vi "Simple SeqProcessor.vi"() -> ()   [LabVIEW 2016, in "SeqProcessor.lvlib"]
uses:
  SeqProcessor.lvlib
  controls/StepScript.ctl
  controls/StepType.ctl
  controls/StepResult.ctl
  controls/StepStatus.ctl
  <vilib>/addons/Qbus/Qbus.lvclass
panel:
  out "error out (no error)":errorcluster
  in  "error in (no error)":errorcluster
  in  "Seq":T1[](array[typedef])=[{"Type"=enum."Normal", "Step"=[{"Action"="StepA", "Process"="ProcessB", "Jump"=0, "Data"="", "Condition"=FALSE}]}, {"Type"=enum."Normal", "Step"=[{"Action"="StepB", "Process"="ProcessB", "Jump"=0, "Data"="", "Condition"=FALSE}]}, {"Type"=enum."Normal", "Step"=[{"Action"="StepC", "Process"="ProcessA", "Jump"=0, "Data"="", "Condition"=FALSE}]}]
  in  "Run":bool
  in  "Stop":bool
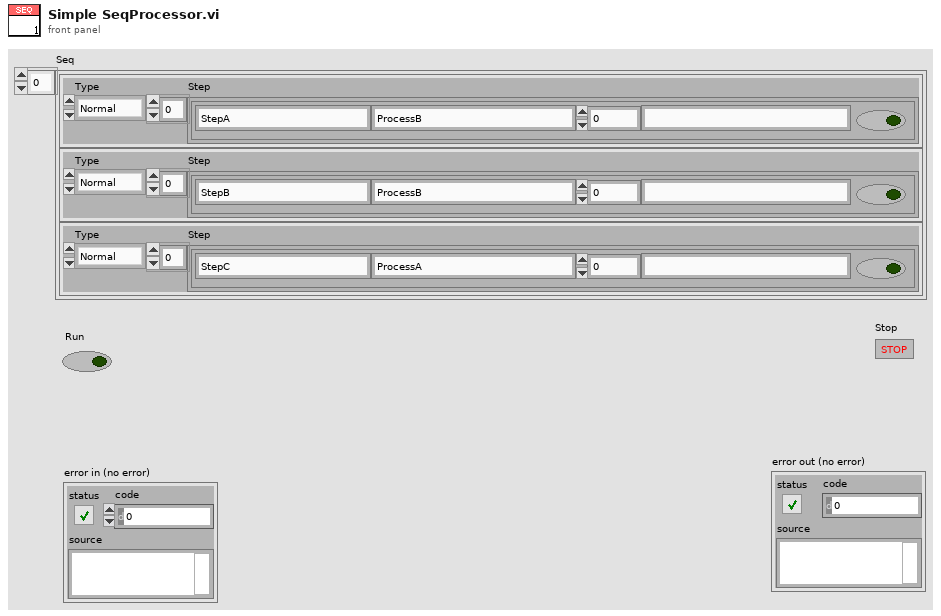
[diagram p1: front panel]
types:
  T1 = typedef "SeqProcessor.lvlib/StepScript.ctl" = cluster{"Type":T2, "Step":cluster{"Action":string, "Process":string, "Jump":i32, "Data":string, "Condition":bool}[]}
  T2 = typedef "SeqProcessor.lvlib/StepType.ctl" = enum16{"Normal", "Parallel", "Conditional", "Jump"}
  T3 = typedef "SeqProcessor.lvlib/StepResult.ctl" = cluster{"Status":T4, "Message":string, "Data":variant}
  T4 = typedef "SeqProcessor.lvlib/StepStatus.ctl" = enum16{"Undone", "Finish", "Error"}
  T5 = typedef "SeqProcessor.lvlib/StepIndex.ctl" = cluster{"Index1":u32, "Index2":u32}
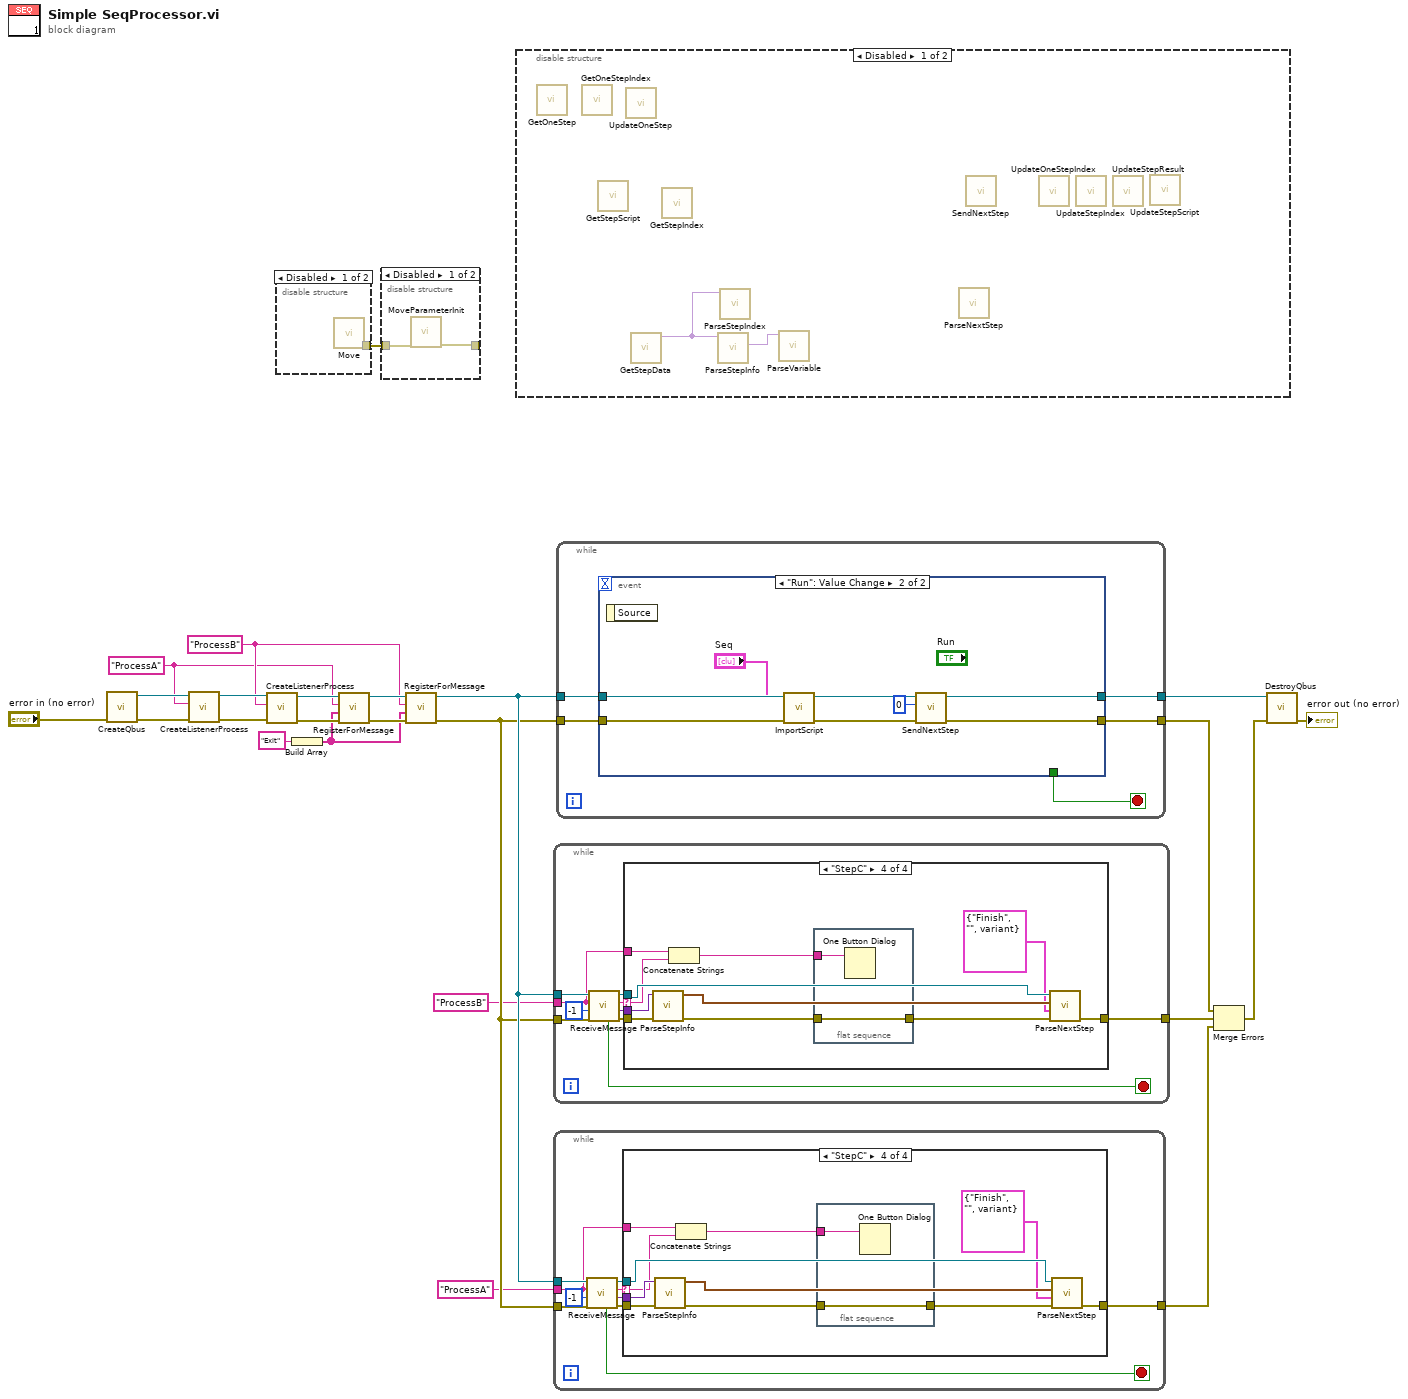
[diagram p0: block diagram]
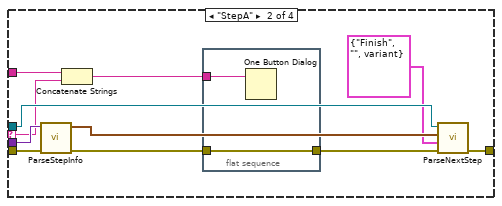
[diagram p3: hidden frame]
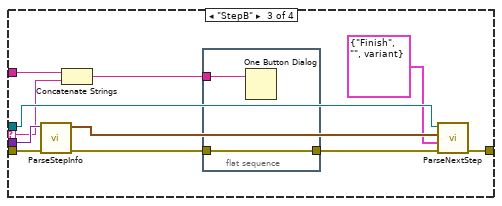
[diagram p4: hidden frame]
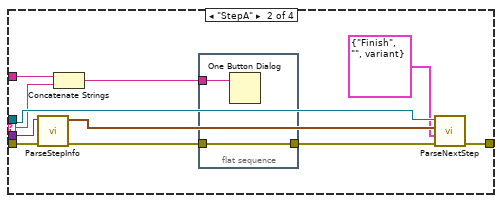
[diagram p6: hidden frame]
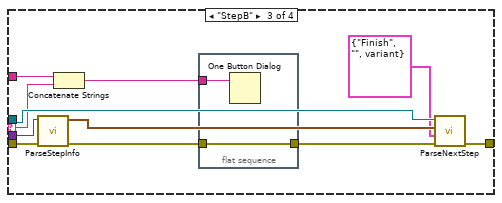
[diagram p7: hidden frame]
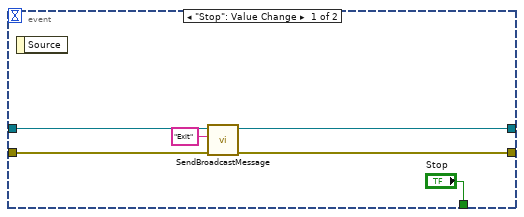
[diagram p8: hidden frame]
diagram:
  w8 = "ProcessB" ("process name")
  w6 = "ProcessA" ("process name")
  n1 = call <vilib>:"CreateQbus.vi"("error in (no error)"="error in (no error)") -> ("error out"=w22:errorcluster, "Qbus"=w23:refnum<class "Qbus.lvclass">)  [unwired: 9 in]
  n2 = call <vilib>:"CreateListenerProcess.vi"("error in (no error)"=w22, "process name"=w6, "Qbus in"=w23) -> ("error in (no error)"=w21:errorcluster, "Qbus out"=w20:refnum<class "Qbus.lvclass">)  [unwired: 7 in]
  n3 = call <vilib>:"CreateListenerProcess.vi"("error in (no error)"=w21, "process name"=w8, "Qbus in"=w20) -> ("error in (no error)"=w15:errorcluster, "Qbus out"=w16:refnum<class "Qbus.lvclass">)  [unwired: 7 in]
  n4 = disable-structure shown="Disabled" {
    disable-tunnel: [w25 _] -> w24
    frame Disabled {
      n5 = call "Move.vi"() -> ("error out"=w25:errorcluster)  [unwired: 11 in]
    }
    frame Enabled {
    }
  }
  n6 = Build Array("Exit" ("message name")) -> (w9:string[])
  n7 = call <vilib>:"RegisterForMessage.vi"("error in (no error)"=w15, "message names"=w9, "process name"=w6, "Qbus in"=w16) -> ("error in (no error)"=w13:errorcluster, "Qbus out"=w14:refnum<class "Qbus.lvclass">)  [unwired: 6 in]
  n8 = disable-structure shown="Disabled" {
    disable-tunnel: w24 -> [w27 w28]
    disable-tunnel: [w26 w28] -> _
    frame Disabled {
      n9 = call "MoveParameterInit.vi"("error in (no error)"=w27) -> ("Error Out"=w26:errorcluster)  [unwired: 10 in]
    }
    frame Enabled {
    }
  }
  n10 = call <vilib>:"RegisterForMessage.vi"("error in (no error)"=w13, "message names"=w9, "process name"=w8, "Qbus in"=w14) -> ("error in (no error)"=w11:errorcluster, "Qbus out"=w12:refnum<class "Qbus.lvclass">)  [unwired: 6 in]
  n11 = disable-structure shown="Disabled" {
    frame Disabled {
      n12 = call "GetOneStep.vi"() -> ()  [unwired: 9 in, 3 out]
      n13 = call "GetOneStepIndex.vi"() -> ()  [unwired: 9 in, 3 out]
      n14 = call "GetStepScript.vi"() -> ()  [unwired: 9 in, 3 out]
      n15 = call "UpdateOneStep.vi"() -> ()  [unwired: 11 in, 1 out]
      n16 = call "GetStepData.vi"() -> ("Data"=w29:variant)  [unwired: 9 in, 2 out]
      n17 = call "GetStepIndex.vi"() -> ()  [unwired: 9 in, 3 out]
      n18 = call "ParseStepInfo.vi"("Data"=w29) -> ("StepData"=w30:variant)  [unwired: 7 in, 3 out]
      n19 = call "ParseStepIndex.vi"("Data"=w29) -> ()  [unwired: 9 in, 2 out]
      n20 = call "ParseVariable.vi"("Variant"=w30) -> ()  [unwired: 8 in, 3 out]
      n21 = call "ParseNextStep.vi"() -> ()  [unwired: 11 in, 1 out]
      n22 = call "SendNextStep.vi"() -> ()  [unwired: 11 in, 1 out]
      n23 = call "UpdateOneStepIndex.vi"() -> ()  [unwired: 9 in, 3 out]
      n24 = call "UpdateStepIndex.vi"() -> ()  [unwired: 11 in, 1 out]
      n25 = call "UpdateStepResult.vi"() -> ()  [unwired: 10 in, 2 out]
      n26 = call "UpdateStepScript.vi"() -> ()  [unwired: 11 in, 1 out]
    }
    frame Enabled {
    }
  }
  n27 = while {
    tunnel: w12 -> [w39]
    tunnel: w11 -> [w40]
    tunnel: "ProcessB" ("process name") -> [w31]
    tunnel: [w32] -> w18
    stop <- w34 stop-if-true
    n28 = call <vilib>:"ReceiveMessage.vi"("error in (no error)"=w40, "timeout (0)"=-1, "process name"=w31, "Qbus in"=w39) -> ("error in (no error)"=w35:errorcluster, "message value"=w36:variant, "message name"=w37:string, "Qbus out"=w38:refnum<class "Qbus.lvclass">, "exit"=w34:bool)  [unwired: 2 in, 1 out]
    n29 = case shown="\"StepC\"" w37 {
      selector: w37 -> [_ w45 w58 w71]
      tunnel: w38 -> [_ w49 w62 w75]
      tunnel: w36 -> [_ w51 w64 w77]
      tunnel: w35 -> [w41 w52 w65 w78]
      tunnel: [w41 w48 w61 w74] -> w32
      tunnel: w31 -> [_ w46 w59 w72]
      frame "", Default {
      }
      frame "StepA" {
        n30 = call "ParseStepInfo.vi"("error in (no error)"=w52, "Data"=w51) -> ("error out"=w43:errorcluster, "StepIndex"=w50:T5)  [unwired: 6 in, 2 out]
        n31 = Concatenate Strings(w46, w45) -> (w44:string)
        n32 = flat-sequence {
          tunnel: w44 -> [w54]
          tunnel: w43 -> [w53]
          tunnel: [w53] -> w42
          frame #0 {
            n33 = One Button Dialog(message=w54) -> ()  [unwired: 1 in, 1 out]
          }
        }
        n34 = call "ParseNextStep.vi"("error in (no error)"=w42, "Result"=T3 {"Status"=enum."Finish", "Message"="", "Data"=variant}, "Index"=w50, "Qbus in"=w49) -> ("error out"=w48:errorcluster)  [unwired: 7 in]
      }
      frame "StepB" {
        n35 = call "ParseStepInfo.vi"("error in (no error)"=w65, "Data"=w64) -> ("error out"=w56:errorcluster, "StepIndex"=w63:T5)  [unwired: 6 in, 2 out]
        n36 = Concatenate Strings(w59, w58) -> (w57:string)
        n37 = flat-sequence {
          tunnel: w57 -> [w67]
          tunnel: w56 -> [w66]
          tunnel: [w66] -> w55
          frame #0 {
            n38 = One Button Dialog(message=w67) -> ()  [unwired: 1 in, 1 out]
          }
        }
        n39 = call "ParseNextStep.vi"("error in (no error)"=w55, "Result"=T3 {"Status"=enum."Finish", "Message"="", "Data"=variant}, "Index"=w63, "Qbus in"=w62) -> ("error out"=w61:errorcluster)  [unwired: 7 in]
      }
      frame "StepC" {
        n40 = call "ParseStepInfo.vi"("error in (no error)"=w78, "Data"=w77) -> ("error out"=w69:errorcluster, "StepIndex"=w76:T5)  [unwired: 6 in, 2 out]
        n41 = Concatenate Strings(w72, w71) -> (w70:string)
        n42 = flat-sequence {
          tunnel: w70 -> [w80]
          tunnel: w69 -> [w79]
          tunnel: [w79] -> w68
          frame #0 {
            n43 = One Button Dialog(message=w80) -> ()  [unwired: 1 in, 1 out]
          }
        }
        n44 = call "ParseNextStep.vi"("error in (no error)"=w68, "Result"=T3 {"Status"=enum."Finish", "Message"="", "Data"=variant}, "Index"=w76, "Qbus in"=w75) -> ("error out"=w74:errorcluster)  [unwired: 7 in]
      }
    }
  }
  n45 = while {
    tunnel: w12 -> [w89]
    tunnel: w11 -> [w90]
    tunnel: "ProcessA" ("process name") -> [w81]
    tunnel: [w82] -> w4
    stop <- w84 stop-if-true
    n46 = call <vilib>:"ReceiveMessage.vi"("error in (no error)"=w90, "timeout (0)"=-1, "process name"=w81, "Qbus in"=w89) -> ("error in (no error)"=w85:errorcluster, "message value"=w86:variant, "message name"=w87:string, "Qbus out"=w88:refnum<class "Qbus.lvclass">, "exit"=w84:bool)  [unwired: 2 in, 1 out]
    n47 = case shown="\"StepC\"" w87 {
      selector: w87 -> [_ w94 w107 w120]
      tunnel: w88 -> [_ w99 w112 w125]
      tunnel: w86 -> [_ w100 w113 w126]
      tunnel: w85 -> [w91 w101 w114 w127]
      tunnel: [w91 w98 w111 w124] -> w82
      tunnel: w81 -> [_ w95 w108 w121]
      frame "", Default {
      }
      frame "StepA" {
        n48 = call "ParseStepInfo.vi"("error in (no error)"=w101, "Data"=w100) -> ("error out"=w93:errorcluster, "StepIndex"=w102:T5)  [unwired: 6 in, 2 out]
        n49 = Concatenate Strings(w95, w94) -> (w96:string)
        n50 = flat-sequence {
          tunnel: w96 -> [w104]
          tunnel: w93 -> [w103]
          tunnel: [w103] -> w92
          frame #0 {
            n51 = One Button Dialog(message=w104) -> ()  [unwired: 1 in, 1 out]
          }
        }
        n52 = call "ParseNextStep.vi"("error in (no error)"=w92, "Result"=T3 {"Status"=enum."Finish", "Message"="", "Data"=variant}, "Index"=w102, "Qbus in"=w99) -> ("error out"=w98:errorcluster)  [unwired: 7 in]
      }
      frame "StepB" {
        n53 = call "ParseStepInfo.vi"("error in (no error)"=w114, "Data"=w113) -> ("error out"=w106:errorcluster, "StepIndex"=w115:T5)  [unwired: 6 in, 2 out]
        n54 = Concatenate Strings(w108, w107) -> (w109:string)
        n55 = flat-sequence {
          tunnel: w109 -> [w117]
          tunnel: w106 -> [w116]
          tunnel: [w116] -> w105
          frame #0 {
            n56 = One Button Dialog(message=w117) -> ()  [unwired: 1 in, 1 out]
          }
        }
        n57 = call "ParseNextStep.vi"("error in (no error)"=w105, "Result"=T3 {"Status"=enum."Finish", "Message"="", "Data"=variant}, "Index"=w115, "Qbus in"=w112) -> ("error out"=w111:errorcluster)  [unwired: 7 in]
      }
      frame "StepC" {
        n58 = call "ParseStepInfo.vi"("error in (no error)"=w127, "Data"=w126) -> ("error out"=w119:errorcluster, "StepIndex"=w128:T5)  [unwired: 6 in, 2 out]
        n59 = Concatenate Strings(w121, w120) -> (w122:string)
        n60 = flat-sequence {
          tunnel: w122 -> [w130]
          tunnel: w119 -> [w129]
          tunnel: [w129] -> w118
          frame #0 {
            n61 = One Button Dialog(message=w130) -> ()  [unwired: 1 in, 1 out]
          }
        }
        n62 = call "ParseNextStep.vi"("error in (no error)"=w118, "Result"=T3 {"Status"=enum."Finish", "Message"="", "Data"=variant}, "Index"=w128, "Qbus in"=w125) -> ("error out"=w124:errorcluster)  [unwired: 7 in]
      }
    }
  }
  n63 = while {
    tunnel: w12 -> [w135]
    tunnel: w11 -> [w134]
    tunnel: [w132] -> w19
    tunnel: [w131] -> w3
    stop <- w133 stop-if-true
    n64 = event shown="[1] \"Run\": Value Change" {
      selector: _ -> [_ _]
      dyn-events: _ -> [_ _]
      timeout: _ -> [_ _]
      tunnel: w135 -> [w140 w144]
      tunnel: w134 -> [w139 w147]
      tunnel: ["Stop" _] -> w133
      tunnel: [w137 w144] -> w132
      tunnel: [w136 w143] -> w131
      event "Stop": Value Change {
        n65 = event-data() -> ()  [unwired: 1 in, 1 out]
        n66 = call <vilib>:"SendBroadcastMessage.vi"("error in (no error)"=w139, "message name"="Exit", "Qbus in"=w140) -> ("error in (no error)"=w136:errorcluster, "Qbus out"=w137:refnum<class "Qbus.lvclass">)  [unwired: 7 in]
      }
      event "Run": Value Change {
        n67 = event-data() -> ()  [unwired: 1 in, 1 out]
        n68 = call "ImportScript.vi"("error in (no error)"=w147, "Seq"="Seq") -> ("error out"=w146:errorcluster)  [unwired: 9 in]
        n69 = call "SendNextStep.vi"("error in (no error)"=w146, "StepIndex"=u32 0, "Qbus in"=w144) -> ("error out"=w143:errorcluster)  [unwired: 8 in]
      }
    }
  }
  n70 = Merge Errors(w3, w18, w4) -> (w17:errorcluster)
  n71 = call <vilib>:"DestroyQbus.vi"("error in (no error)"=w17, "Qbus"=w19) -> ("error in (no error)"=→"error out (no error)":errorcluster)  [unwired: 9 in]
